vi "IO_MFA_AIN_Set_AdcOffset1.vi"(11 "AdcOffset":sgl) -> (3 "ADC Offset Error":bool)   [LabVIEW 2011]
panel:
  out "error ADC":errorcluster
  out "AAABuild":i32
  in  "MintController":refnum<k7>(container)
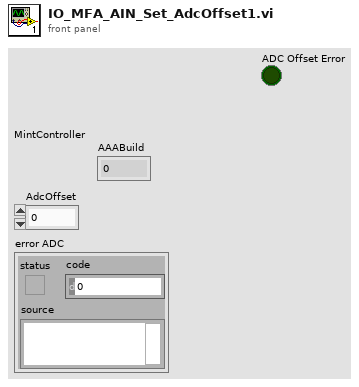
[diagram p1: front panel]
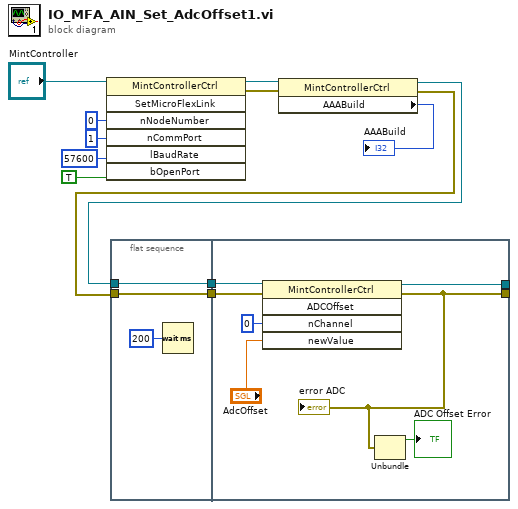
[diagram p0: block diagram]
diagram:
  n1 = invoke class="MintControllerCtrl" method="SetMicroFlexLink"(reference="MintController", "nNodeNumber"=i16 0, "nCommPort"=i16 1, "lBaudRate"=57600, "bOpenPort"=TRUE) -> (reference out=w12:refnum<k7>, error out=w6:errorcluster)  [unwired: 2 in, 5 out]
  n2 = flat-sequence {
    tunnel: [w15] -> w4
    tunnel: [w13] -> w3
    tunnel: w2 -> [w15]
    tunnel: w1 -> [w13]
    tunnel: w4 -> [w22]
    tunnel: w3 -> [w21]
    tunnel: [w17] -> _
    tunnel: [w20] -> _
    frame #0 {
      n3 = Wait (ms)(milliseconds to wait=u32 200) -> ()  [unwired: 1 out]
    }
    frame #1 {
      n4 = invoke class="MintControllerCtrl" method="ADCOffset"(reference=w21, error in=w22, "nChannel"=i16 0, "newValue"="AdcOffset") -> (reference out=w20:refnum<k7>, error out=w17:errorcluster)  [unwired: 1 in, 3 out]
      "error ADC" <- w17
      n5 = Unbundle(w17) -> ("status"=→"ADC Offset Error":bool)  [unwired: 2 out]
    }
  }
  n6 = property class="MintControllerCtrl"(reference=w12, error in=w6) -> (reference out=w1:refnum<k7>, error out=w2:errorcluster, "AAABuild"=→"AAABuild":i32)
